vi "ElevatorBrake.vi"(5 "Elevator Manual Mode":bool, 7 "Manual Movement":dbl, 8 "Feed Forward Contribution":dbl, 9 "Elevator State In":string, 10 "Elevator Power In":dbl, 11 "Elevator Error":dbl) -> (1 "Elevator State Out":string, 2 "Elevator Power Out":dbl)   [LabVIEW 2018]
uses:
  Inputs_DriverStation.vi
  SensorReadings.vi
  RobotStates.vi
panel:
  in  "Brake Pressure Threshold (PSI)":dbl=60.0
  in  "Hysteresis Threshold (ms)":u32=500
  in  "Encoder Check Delay (ms)":u32=1000000
  in  "Time in Error Band (ms)":u32=1000
  in  "Error Band (in)":dbl=20.0
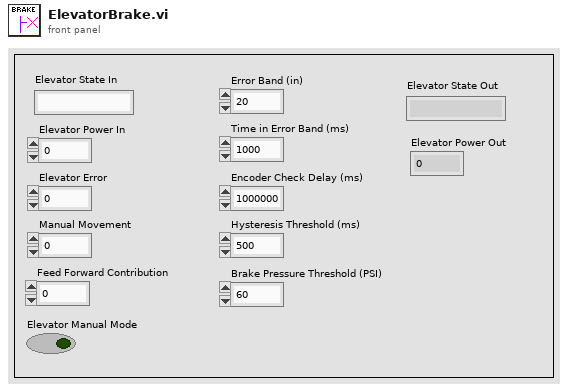
[diagram p1: front panel]
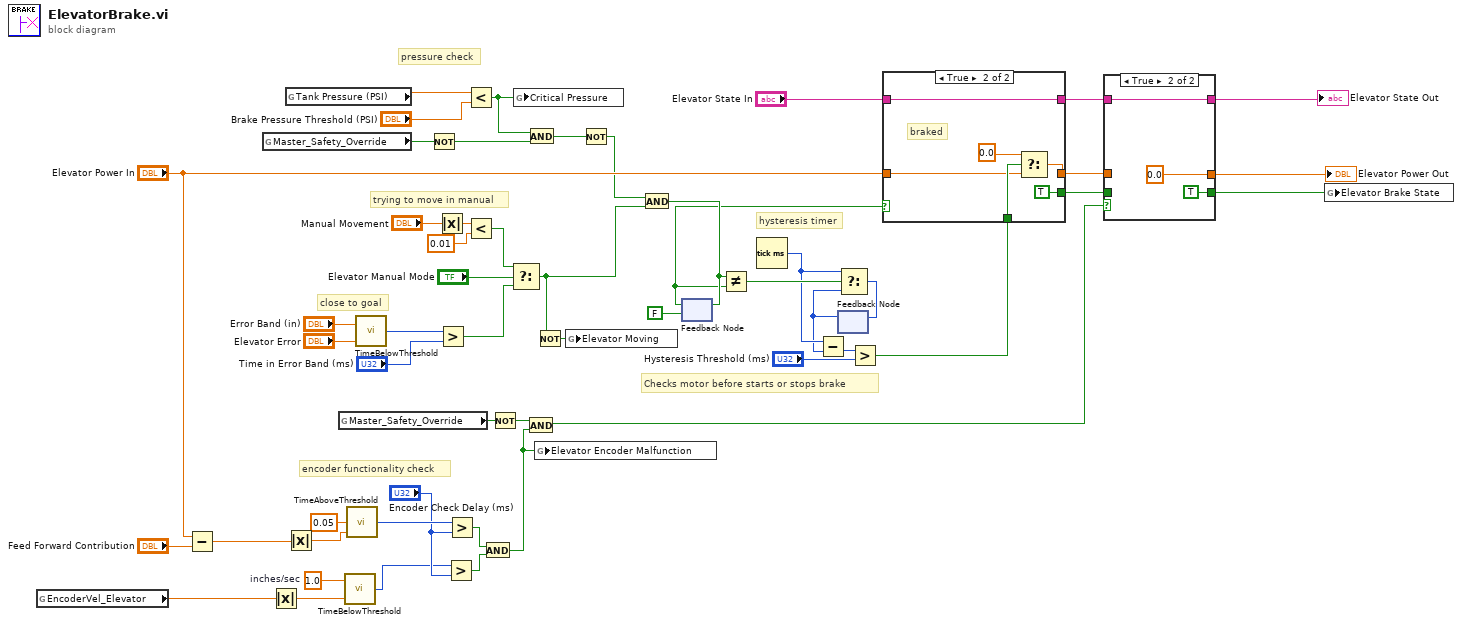
[diagram p0: block diagram]
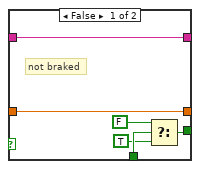
[diagram p3: hidden frame]
diagram:
  w39 = 1.0  # inches/sec
  # "Checks motor before starts or stops brake"
  # "hysteresis timer"
  # "pressure check"
  # "encoder functionality check"
  # "trying to move in manual"
  # "close to goal"
  n1 = global read "SensorReadings.vi" "EncoderVel_Elevator"() -> (w40:dbl)
  n2 = Subtract(x="Elevator Power In", y="Feed Forward Contribution") -> (x-y=w30:dbl)
  n3 = global read "Inputs_DriverStation.vi" "Master_Safety_Override"() -> (w27:bool)
  n4 = Absolute Value(x=w40) -> (abs(x)=w29:dbl)
  n5 = global read "SensorReadings.vi" "Tank Pressure (PSI)"() -> (w7:dbl)
  n6 = Absolute Value(x=w30) -> (abs(x)=w37:dbl)
  n7 = global read "Inputs_DriverStation.vi" "Master_Safety_Override"() -> (w41:bool)
  n8 = call "TimeBelowThreshold.vi"("Current Value"=w29, "Threshold"=w39) -> ("Time Below"=w8:u32)  [unwired: 3 in]
  n9 = call "TimeAboveThreshold.vi"("Current Value"=w37, "Threshold"=0.05) -> ("Time Above"=w36:u32)  [unwired: 3 in]
  n10 = call "TimeBelowThreshold.vi"("Current Value"="Elevator Error", "Threshold"="Error Band (in)") -> ("Time Below"=w51:u32)  [unwired: 3 in]
  n11 = Not(x=w27) -> (.not. x?=w26:bool)
  n12 = Absolute Value(x="Manual Movement") -> (abs(x)=w48:dbl)
  n13 = Greater?(x=w51, y="Time in Error Band (ms)") -> (0:w46:bool)
  n14 = Greater?(x=w8, y="Encoder Check Delay (ms)") -> (0:w34:bool)
  n15 = Greater?(x=w36, y="Encoder Check Delay (ms)") -> (0:w35:bool)
  n16 = Less?(x=w7, y="Brake Pressure Threshold (PSI)") -> (x < y?=w6:bool)
  n17 = Less?(x=w48, y=0.01) -> (x < y?=w44:bool)
  n18 = And(x=w35, y=w34) -> (x .and. y?=w28:bool)
  n19 = Not(x=w41) -> (.not. x?=w42:bool)
  n20 = Select(t=w44, s="Elevator Manual Mode", f=w46) -> (s? t:f=w4:bool)
  n21 = global write "SensorReadings.vi" "Critical Pressure"(w6) -> ()
  n22 = And(x=w42, y=w28) -> (x .and. y?=w9:bool)
  n23 = And(x=w6, y=w26) -> (x .and. y?=w25:bool)
  n24 = Not(x=w4) -> (.not. x?=w3:bool)
  n25 = global write "SensorReadings.vi" "Elevator Encoder Malfunction"(w28) -> ()
  n26 = global write "RobotStates.vi" "Elevator Moving"(w3) -> ()
  n27 = Not(x=w25) -> (.not. x?=w24:bool)
  n28 = And(x=w24, y=w4) -> (x .and. y?=w22:bool)
  n29 = feedback-in #1(w22) -> ()
  n30 = feedback #1(FALSE) -> (w2:bool)
  n31 = Not Equal?(x=w22, y=w2) -> (x != y?=w20:bool)
  n32 = Tick Count (ms)() -> (millisecond timer value=w18:u32)
  n33 = feedback #2() -> (w17:u32)  [unwired: 1 in]
  n34 = Subtract(x=w18, y=w17) -> (x-y=w19:u32)
  n35 = Select(t=w18, s=w20, f=w17) -> (s? t:f=w21:u32)
  n36 = feedback-in #2(w21) -> ()
  n37 = Greater?(x=w19, y="Hysteresis Threshold (ms)") -> (0:w10:bool)
  n38 = case shown="True" w2 {
    tunnel: "Elevator Power In" -> [w59 w60]
    tunnel: [w59 w63] -> w13
    tunnel: [w54 TRUE] -> w15
    tunnel: "Elevator State In" -> [w58 w64]
    tunnel: [w58 w64] -> w12
    tunnel: w10 -> [w57 w61]
    frame False {
      # "not braked"
      n39 = Select(t=FALSE, s=w57, f=TRUE) -> (s? t:f=w54:bool)
    }
    frame True {
      # "braked"
      n40 = Select(t=0.0 ("Elevator Power In"), s=w61, f=w60) -> (s? t:f=w63:dbl)
    }
  }
  n41 = case shown="True" w9 {
    tunnel: [w66 TRUE ("f")] -> w14
    tunnel: w15 -> [w66 _]
    tunnel: [w67 0.0 ("Elevator Power In")] -> w1
    tunnel: w13 -> [w67 _]
    tunnel: [w68 w71] -> w11
    tunnel: w12 -> [w68 w71]
    frame False {
    }
    frame True {
    }
  }
  "Elevator Power Out" <- w1
  "Elevator State Out" <- w11
  n42 = global write "RobotStates.vi" "Elevator Brake State"(w14) -> ()
